vi "Automatischer Wechsel Charts.vi"   [LabVIEW 2020, in "Bildwechsel.lvlib"]
uses:
  Bildwechsel.lvlib
  Bild-Auswahl.ctl
types:
  T1 = typedef "Bildwechsel.lvlib/Bild-Auswahl.ctl" = enum16{"lesen", "Initialisieren", "Beenden", "Grafik", "Anlagenübersicht", "Anlagengrenzwerte", "Log Konfig", "Gaszuordnung AO", "Erw. Konfiguration", "FT-IR  ", "Störmeldungen", "Störmeldepuffer", "Störmeldekonfig", "PNS Grenzwerte", "Statusübersicht", "Linearisierung", "ARN", "EPA Dichtheitstest", "Lin-Nachweis", "FID", "PMA", "CalGas", "Lambda", "Interference", "PNS Chart"}
  T2 = typedef "Bildwechsel.lvlib/Bild-Auswahl.ctl" = enum16{"lesen", "Initialisieren", "Beenden", "Grafik", "Anlagenübersicht", "Anlagengrenzwerte", "Log Konfig", "Gaszuordnung AO", "Erw. Konfiguration", "FT-IR  ", "Störmeldungen", "Störmeldepuffer", "Störmeldekonfig", "PNS Grenzwerte", "Statusübersicht", "Linearisierung", "ARN", "EPA Dichtheitstest", "FID", "PMA", "CalGas", "Lambda", "Interference", "Amium PNS"}
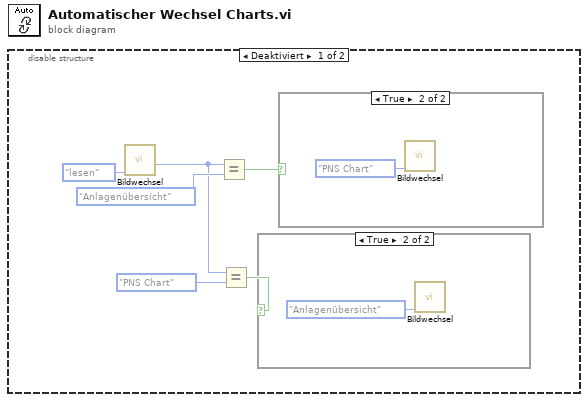
[diagram p0: block diagram]
diagram:
  n1 = disable-structure shown="Deaktiviert" {
    frame Disabled {
      n2 = call "Bildwechsel.vi"("nächstes Bild"=Bild-Auswahl."lesen") -> ("aktuelle Bildnummer"=w3:T2)  [unwired: 9 in, 1 out]
      n3 = Equal?(x=w3, y=Bild-Auswahl."Anlagenübersicht") -> (x = y?=w4:bool)
      n4 = Equal?(x=w3, y=Bild-Auswahl."PNS Chart") -> (x = y?=w1:bool)
      n5 = case shown="True" w1 {
        frame False {
        }
        frame True {
          n6 = call "Bildwechsel.vi"("nächstes Bild"=Bild-Auswahl."Anlagenübersicht") -> ()  [unwired: 9 in, 2 out]
        }
      }
      n7 = case shown="True" w4 {
        frame False {
        }
        frame True {
          n8 = call "Bildwechsel.vi"("nächstes Bild"=Bild-Auswahl."PNS Chart") -> ()  [unwired: 9 in, 2 out]
        }
      }
    }
    frame Enabled {
    }
  }
